vi "Filter for Report.vi"(5 "Report Data Type (Report Data = Disable)":refnum<class "Report Data.lvclass">, 7 "Action class name (\"\" = Disable)":string, 8 "error in (no error)":errorcluster, 9 "Type filter (Report = Disable)":T1=enum."Report", 10 "Action Number(Empty = Disable)":i32[](array[numeric]), 11 "Project Builder in":refnum<class "Project Builder.lvclass">) -> (0 "error out":errorcluster, 1 "Match Found?":bool, 2 "Filtered Reports":refnum<class "Report Data.lvclass">[](array[class]), 3 "Typed Report Data (If type is matched)":refnum<class "Report Data.lvclass">, 4 "Match Count":i32)   [LabVIEW 2019, in "ProjectBuilder.lvlib" / "Project Builder.lvclass"]
doc: "Filter for a desired Result using the VI input."
uses:
  Project Builder.lvclass
  Data/Report Data/Report Data.lvclass
  Ctl/Ctl_Build Steps.ctl
  Project Builder.lvclass/Project Builder.ctl
  Data/Report Data/Report Data.lvclass/Report Data.ctl
  Project Action/Project Action.lvclass/Project Action.ctl
  Project Action/Project Action.lvclass
  PPL/HDH.ClassLoader.lvlibp
  ProjectBuilder.lvlib
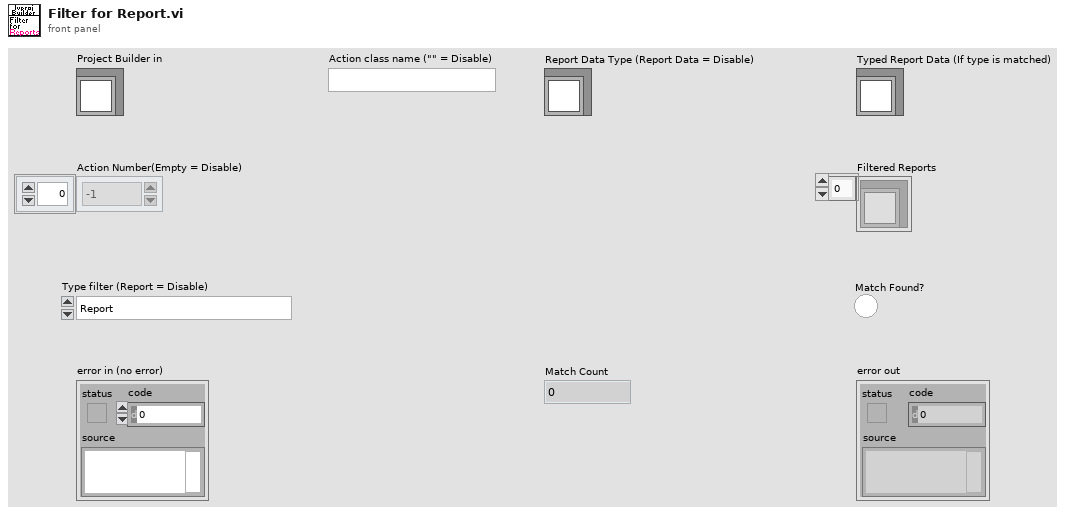
[diagram p1: front panel]
types:
  T1 = typedef "ProjectBuilder.lvlib/Ctl_Build Steps.ctl" = enum16{"Source Test", "Build", "Post-Build Test", "Deploy", "Report"}
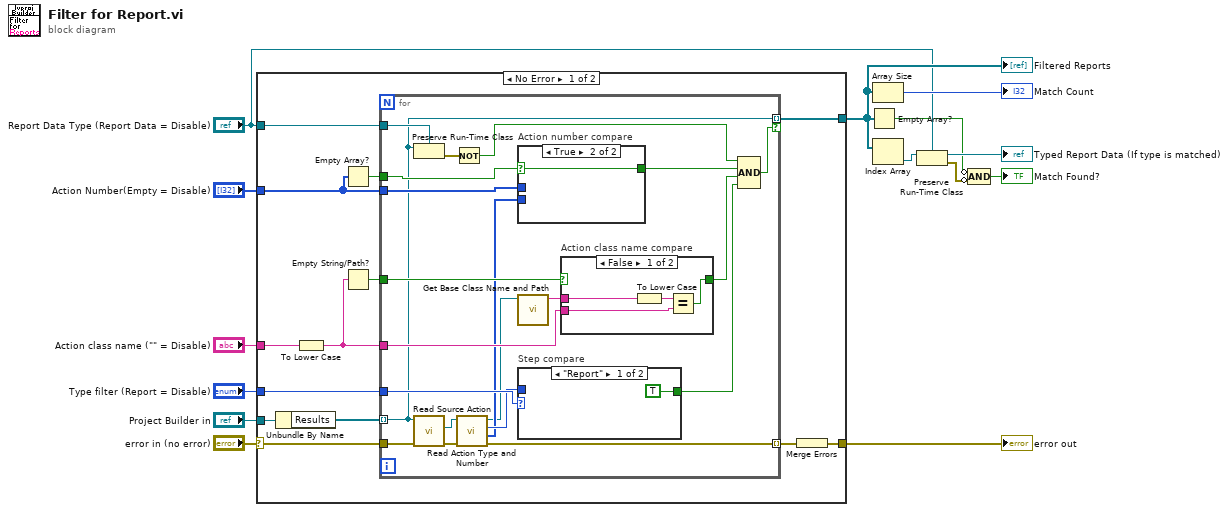
[diagram p0: block diagram]
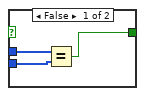
[diagram p2: hidden frame]
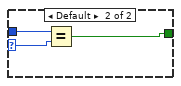
[diagram p3: hidden frame]
diagram:
  n1 = case shown="No Error" "error in (no error)" {
    selector: "error in (no error)" -> [w20 w62]
    tunnel: [w15 w62] -> w13
    tunnel: "Project Builder in" -> [w27 _]
    tunnel: "Action class name (\"\" = Disable)" -> [w25 _]
    tunnel: [w22 _] -> w7
    tunnel: "Type filter (Report = Disable)" -> [w21 _]
    tunnel: "Action Number(Empty = Disable)" -> [w17 _]
    tunnel: "Report Data Type (Report Data = Disable)" -> [w16 _]
    frame No Error {
      n2 = Unbundle By Name(w27) -> ("Results"=w26:refnum<class "Report Data.lvclass">[])
      n3 = To Lower Case(string=w25) -> (all lower case string=w24:string)
      n4 = Empty Array?(array=w17) -> (empty?=w18:bool)
      n5 = Empty String/Path?(string/path=w24) -> (empty?=w23:bool)
      n6 = for {
        tunnel: w26 -> [w33] mode=indexing
        tunnel: w24 -> [w47]
        tunnel: w23 -> [w48]
        tunnel: [w33] -> w22 mode=indexing if=w45
        tunnel: w21 -> [w44]
        tunnel: w18 -> [w42]
        tunnel: w17 -> [w40]
        tunnel: w16 -> [w34]
        tunnel: w20 -> [w29]
        tunnel: [w28] -> w19 mode=indexing
        n7 = Preserve Run-Time Class(object in=w33, 2:w34) -> (error out=w32:errorcluster)  [unwired: 1 in, 1 out]
        n8 = call "Read Source Action.vi"("error in (no error)"=w29, "Report Data in"=w33) -> ("error out"=w30:errorcluster, "Source Action"=w39:refnum<class "Project Action.lvclass">)  [unwired: 7 in, 1 out]
        n9 = Not(x=w32) -> (.not. x?=w31:bool)
        n10 = call "Read Action Type and Number.vi"("error in (no error)"=w30, "Project Action in"=w39) -> ("error out"=w28:errorcluster, "Action Number"=w37:i32[], "Build Step"=w38:T1, "Project Action out"=w36:refnum<class "Project Action.lvclass">)  [unwired: 6 in]
        n11 = case "Action number compare" shown="True" w42 {
          selector: w42 -> [_ w52]
          tunnel: [w49 w52] -> w41
          tunnel: w40 -> [w51 _]
          tunnel: w37 -> [w50 _]
          frame False {
            n12 = Equal?(x=w51, y=w50) -> (x = y?=w49:bool)
          }
          frame True {
          }
        }
        n13 = call "Get Base Class Name and Path.vi"("Class"=w36) -> ("Base Class Name"=w35:string)  [unwired: 8 in, 2 out]
        n14 = case "Step compare" shown="\"Report\"" w44 {
          selector: w44 -> [_ w56]
          tunnel: [TRUE w55] -> w43
          tunnel: w38 -> [_ w54]
          frame "Report" {
          }
          frame Default {
            n15 = Equal?(x=w54, y=w56) -> (x = y?=w55:bool)
          }
        }
        n16 = case "Action class name compare" shown="False" w48 {
          selector: w48 -> [_ w61]
          tunnel: w35 -> [w60 _]
          tunnel: w47 -> [w58 _]
          tunnel: [w57 w61] -> w46
          frame False {
            n17 = To Lower Case(string=w60) -> (all lower case string=w59:string)
            n18 = Equal?(x=w59, y=w58) -> (x = y?=w57:bool)
          }
          frame True {
          }
        }
        n19 = Compound Arithmetic op=AND(w31, w41, w46, w43) -> (w45:bool)
      }
      n20 = Merge Errors(w19) -> (w15:errorcluster)
    }
    frame Error {
    }
  }
  "error out" <- w13
  "Filtered Reports" <- w7
  n21 = Empty Array?(array=w7) -> (empty?=w3:bool)
  n22 = Array Size(array=w7) -> (size(s)=→"Match Count":i32)
  n23 = Index Array(array=w7) -> (element=w6:refnum<class "Report Data.lvclass">)  [unwired: 1 in]
  n24 = Preserve Run-Time Class(object in=w6, 2:"Report Data Type (Report Data = Disable)") -> (object out=→"Typed Report Data (If type is matched)":refnum<class "Report Data.lvclass">, error out=w2:errorcluster)  [unwired: 1 in]
  n25 = Compound Arithmetic op=AND(invert w3, invert w2) -> (→"Match Found?":bool)
